vi "Get FPGA Name from Script.vi"(1 "file":path, 4 "Kasli":refnum<class "Kasli.lvclass">) -> (0 "Kasli Name":string)   [LabVIEW 2020, in "Kasli Wrapper 2.0.lvlib" / "Kasli.lvclass"]
uses:
  Kasli.lvclass
  <vilib>/regexp/Match Regular Expression.xnode
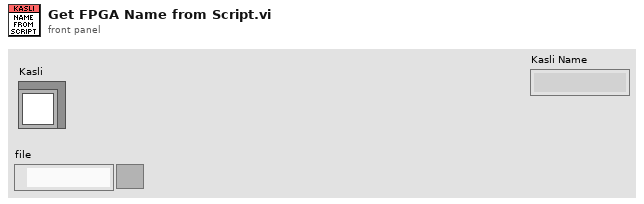
[diagram p1: front panel]
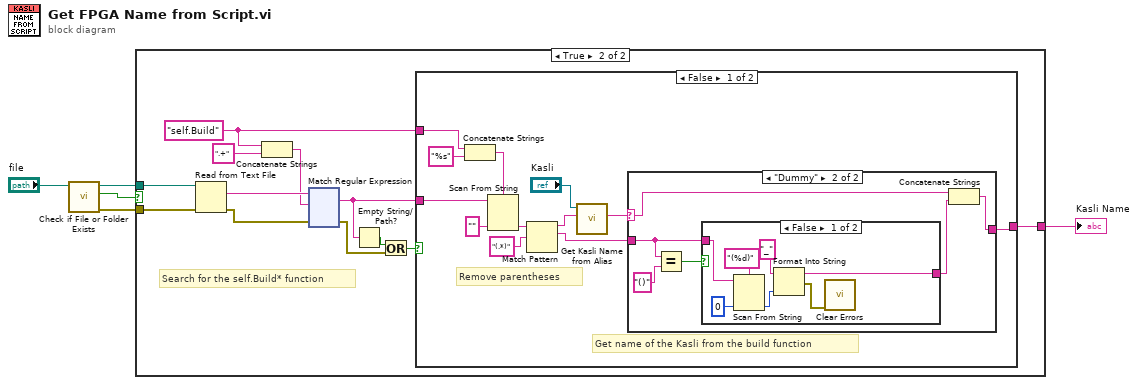
[diagram p0: block diagram]
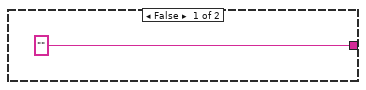
[diagram p2: hidden frame]
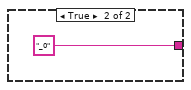
[diagram p4: hidden frame]
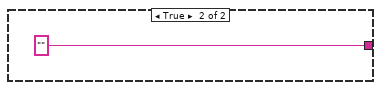
[diagram p5: hidden frame]
diagram:
  n1 = call <vilib>:"Check if File or Folder Exists.vi"("path"="file") -> ("error out"=w1:errorcluster, "file or folder exists?"=w4:bool, "dup path"=w3:path)  [unwired: 8 in]
  n2 = case shown="True" w4 {
    tunnel: w3 -> [_ w14]
    tunnel: ["" ("result string") w13] -> w2
    tunnel: w1 -> [_ w7]
    frame False {
    }
    frame True {
      w15 = "self.Build" ("format string")
      # "Search for the self.Build* function"
      n3 = Read from Text File(file (use dialog)=w14, error in=w7) -> (text=w18:string, error out=w11:errorcluster)  [unwired: 2 in, 2 out]
      n4 = Concatenate Strings(w15, ".+" ("string")) -> (w16:string)
      n5 = xnode "Match Regular Expression"("input string"=w18, "regular expression"=w16, "error in"=w11) -> ("whole match"=w12:string, "error out"=w8:errorcluster)  [unwired: 3 in, 3 out]
      n6 = Empty String/Path?(string/path=w12) -> (empty?=w10:bool)
      n7 = Or(x=w10, y=w8) -> (x .or. y?=w9:bool)
      n8 = case shown="False" w9 {
        tunnel: w12 -> [w30 _]
        tunnel: w15 -> [w27 _]
        tunnel: [w25 "" ("result string")] -> w13
        frame False {
          # "Get name of the Kasli from the build function"
          # "Remove parentheses"
          n9 = Concatenate Strings(w27, "%s" ("string")) -> (w26:string)
          n10 = Scan From String(format string=w26, input string=w30, default 1="" ("default value 1")) -> (output 1=w24:string)  [unwired: 2 in, 3 out]
          n11 = Match Pattern(string=w24, regular expression="(.*)" ("search string")) -> (before substring=w19:string, match substring=w22:string)  [unwired: 1 in, 2 out]
          n12 = call-dynamic "Get Kasli Name from Alias.vi"("Kasli Alias"=w19, "Kasli in"="Kasli") -> ("Kasli Name"=w21:string)  [unwired: 7 in, 2 out]
          n13 = case shown="\"Dummy\"" w21 {
            selector: w21 -> [w31 w37]
            tunnel: [w31 w36] -> w25
            tunnel: w22 -> [_ w34]
            frame Default {
            }
            frame "Dummy" {
              n14 = Equal?(x=w34, y="()") -> (x = y?=w32:bool)
              n15 = case shown="False" w32 {
                tunnel: w34 -> [w42 _]
                tunnel: [w40 "_0"] -> w35
                frame False {
                  n16 = Scan From String(format string="(%d)", input string=w42, default 1=0 ("default value 1")) -> (output 1=w41:i32)  [unwired: 2 in, 3 out]
                  n17 = Format Into String(initial string="_" ("string"), w41) -> (resulting string=w40:string, error out=w38:errorcluster)  [unwired: 2 in]
                  n18 = call <vilib>:"Clear Errors.vi"("error in (no error)"=w38) -> ()  [unwired: 5 in, 2 out]
                }
                frame True {
                }
              }
              n19 = Concatenate Strings(w37, w35) -> (w36:string)
            }
          }
        }
        frame True {
        }
      }
    }
  }
  "Kasli Name" <- w2
